vi "Begin.vi"(8 "error in":errorcluster) -> (0 "error out":errorcluster)   [LabVIEW 2019]
doc: "Called before other user functions, this VI is expected to open initial I/O refnums, load in file data, and do all program initialization. Notice that the <B>error out</B> terminal is simply used for data flow. Wiring it to other structures or subVIs ensures that this VI runs first."
uses:
  <vilib>/Rock Robotics/WPI/DriverStation/WPI_DriverStationRobotMode2.ctl
  Subsystems/Drive/Drive_Cluster.ctl
  Subsystems/Drive/Drive_States.ctl
  Subsystems/Intake/Intake_Cluster.ctl
  Subsystems/Intake/Intake_States.ctl
  Subsystems/Turret/Turret_Cluster.ctl
  Subsystems/Turret/Turret_States.ctl
  Subsystems/Magazine/Magazine_Cluster.ctl
  Subsystems/Magazine/Magazine_States.ctl
  Subsystems/Climb/Climb_Cluster.ctl
  Subsystems/Climb/Climb_States.ctl
  Subsystems/Control_Panel/Control_Panel_Cluster.ctl
  Subsystems/Control_Panel/Control_Panel_States.ctl
  <vilib>/Rock Robotics/WPI/Joystick/WPI_JoystickDeviceEnum.ctl
  <vilib>/Rock Robotics/WPI/ThirdParty/Phoenix-LabVIEW/Motor Controller/Controls/CTRE_Phoenix_MotorControl_ControlMode.ctl
  <vilib>/Rock Robotics/WPI/ThirdParty/REV Robotics/SPARK MAX/Typedef/Spark MAX Control Type.ctl
  Subsystems/Flywheel/Flywheel_Cluster.ctl
  Subsystems/Flywheel/Flywheel_States.ctl
  Robot Global Data.vi
  Globals/Drive_Globals.vi
  Globals/Intake_Globals.vi
  Globals/Turret_Globals.vi
  Globals/Magazine_Globals.vi
  Globals/Climb_Globals.vi
  Globals/Control_Panel_Globals.vi
  Globals/Joystick_Globals.vi
  Globals/Flywheel_Globals.vi
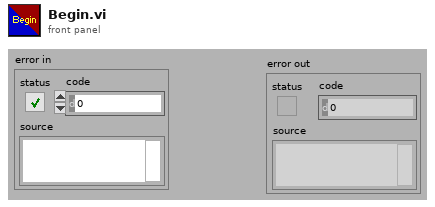
[diagram p1: front panel]
types:
  T1 = typedef "Spark MAX Control Type.ctl" = enum16{"Percent VBus", "Voltage", "Velocity", "Position", "Smart Motion", "Current", "Smart Velocity"}
  T2 = cluster{"P Gain":dbl, "I Gain":dbl, "D Gain":dbl, "F Gain":dbl, "I Zone":dbl, "Min Output":dbl, "Max Output":dbl}
  T3 = typedef "Flywheel_Cluster.ctl" = cluster{"Flywheel_Throttle":dbl, "Control_States":T4, "Auto_Speed":bool, "Flywheel_On":bool}
  T4 = typedef "Flywheel_States.ctl" = enum16{"No-Op", "Percent_Voltage", "Speed_Control_Manual", "Speed_Control_Auto"}
  T5 = typedef "CTRE_Phoenix_MotorControl_ControlMode.ctl" = u16
  T6 = typedef "WPI_JoystickDeviceEnum.ctl" = enum16{"USB 0", "USB 1", "USB 2", "USB 3", "USB 4", "USB 5"}
  T7 = typedef "Control_Panel_Cluster.ctl" = cluster{"Control_State":T8, "Start_Movement":bool, "Abort":bool, "Rotation_Control?":bool, "Positional_Control? ":bool, "Throttle":dbl}
  T8 = typedef "Control_Panel_States.ctl" = enum16{"No-Op", "Rotational_Control", "Positional_Control", "Manual_Control"}
  T9 = typedef "Climb_Cluster.ctl" = cluster{"Control_State":T10, "Extend_Climber?":bool, "Clamp?":bool, "Balance?":bool, "Transverse_Throttle":dbl, "Elevator_Throttle":dbl, "Control_Panel_Setpoint?":bool, "Auto-Balance":bool, "Pivot_Throttle":dbl}
  T10 = typedef "Climb_States.ctl" = enum16{"No-Op", "Extending", "Clamping", "Balancing", "Manual_Control"}
  T11 = typedef "Magazine_Cluster.ctl" = cluster{"Control_States":T12, "Fire":bool, "Magazine_Throttle":dbl}
  T12 = typedef "Magazine_States.ctl" = enum16{"No-Op", "Loading", "Fire", "Unjam", "Manual"}
  T13 = typedef "Turret_Cluster.ctl" = cluster{"Auto-Target?":bool, "Control_State":T14, "Turret_Spin_Speed":dbl, "Turret_Spin_Speed_Control?":bool}
  T14 = typedef "Turret_States.ctl" = enum16{"Manual_Percent_Voltage", "Manual_Speed_Control", "Auto-Target"}
  T15 = typedef "Intake_Cluster.ctl" = cluster{"Control_State":T16, "Intake_On":bool, "Intake_Extended":bool, "Intake_Throttle":dbl}
  T16 = typedef "Intake_States.ctl" = enum16{"Manual_Control"}
  T17 = typedef "Drive_Cluster.ctl" = cluster{"Control_State":T18, "Angular_Throttle":dbl, "Linear_Throttle":dbl, "Torque_Changing":bool}
  T18 = typedef "Drive_States.ctl" = enum16{"Percent_Voltage_Control", "Speed_Control"}
  T19 = typedef "WPI_DriverStationRobotMode2.ctl" = enum16{"Autonomous Disabled", "Autonomous Enabled", "Teleop Disabled", "Teleop Enabled", "Disconnected", "Finish", "Test Disabled", "Test Enabled", "Emergency Stopped"}
  T20 = typedef "WPI_JoystickDevRef.ctl" = cluster{"Device":T6}
  T21 = typedef "WPI_MotorControlDeviceRef.ctl" = cluster{"DeviceStatus":errorcluster, "Type":T22, "PWM":cluster{"PWM Channel":T23, "DeadBand":T24}, "CAN":cluster{"Device Number":u8, "SetOutput VI Ref":variant, "GetOutput VI Ref":variant, "Enable VI Ref":variant, "Disable VI Ref":variant, "Data":variant}, "Invert":bool, "DIO PWM":cluster{"PWM \"Enable\" Channel":T23, "DIOChannel":T25, "PWM Rate":dbl}}
  T22 = typedef "WPI_MotorControlType.ctl" = enum16{"PWM", "CAN", "DIO PWM"}
  T23 = typedef "FPGA_DIOPWMChannel.ctl" = enum8{"PWM 0", "PWM 1", "PWM 2", "PWM 3", "PWM 4", "PWM 5", "PWM 6", "PWM 7", "PWM 8", "PWM 9", "PWM MXP 0", "PWM MXP 1", "PWM MXP 2", "PWM MXP 3", "PWM MXP 4", "PWM MXP 5", "PWM MXP 6", "PWM MXP 7", "PWM MXP 8", "PWM MXP 9", "Invalid"}
  T24 = typedef "WPI_PWMDeadband.ctl" = cluster{"Name":string, "maxPositivePwm":i32, "minPositivePwm":i32, "centerPwm":i32, "maxNegativePwm":i32, "minNegativePwm":i32, "angularRange":u16}
  T25 = typedef "FPGA_DIOChannel.ctl" = enum8{"DIO 0", "DIO 1", "DIO 2", "DIO 3", "DIO 4", "DIO 5", "DIO 6", "DIO 7", "DIO 8", "DIO 9", "DIO MXP 0", "DIO MXP 1", "DIO MXP 2", "DIO MXP 3", "DIO MXP 4", "DIO MXP 5", "DIO MXP 6", "DIO MXP 7", "DIO MXP 8", "DIO MXP 9", "DIO MXP 10", "DIO MXP 11", "DIO MXP 12", "DIO MXP 13", "DIO MXP 14", "DIO MXP 15", "SPI Port CS1", "SPI Port CS2", "SPI Port CS3", "SPI Port MISO", "SPI Port MOSI", "Invalid"}
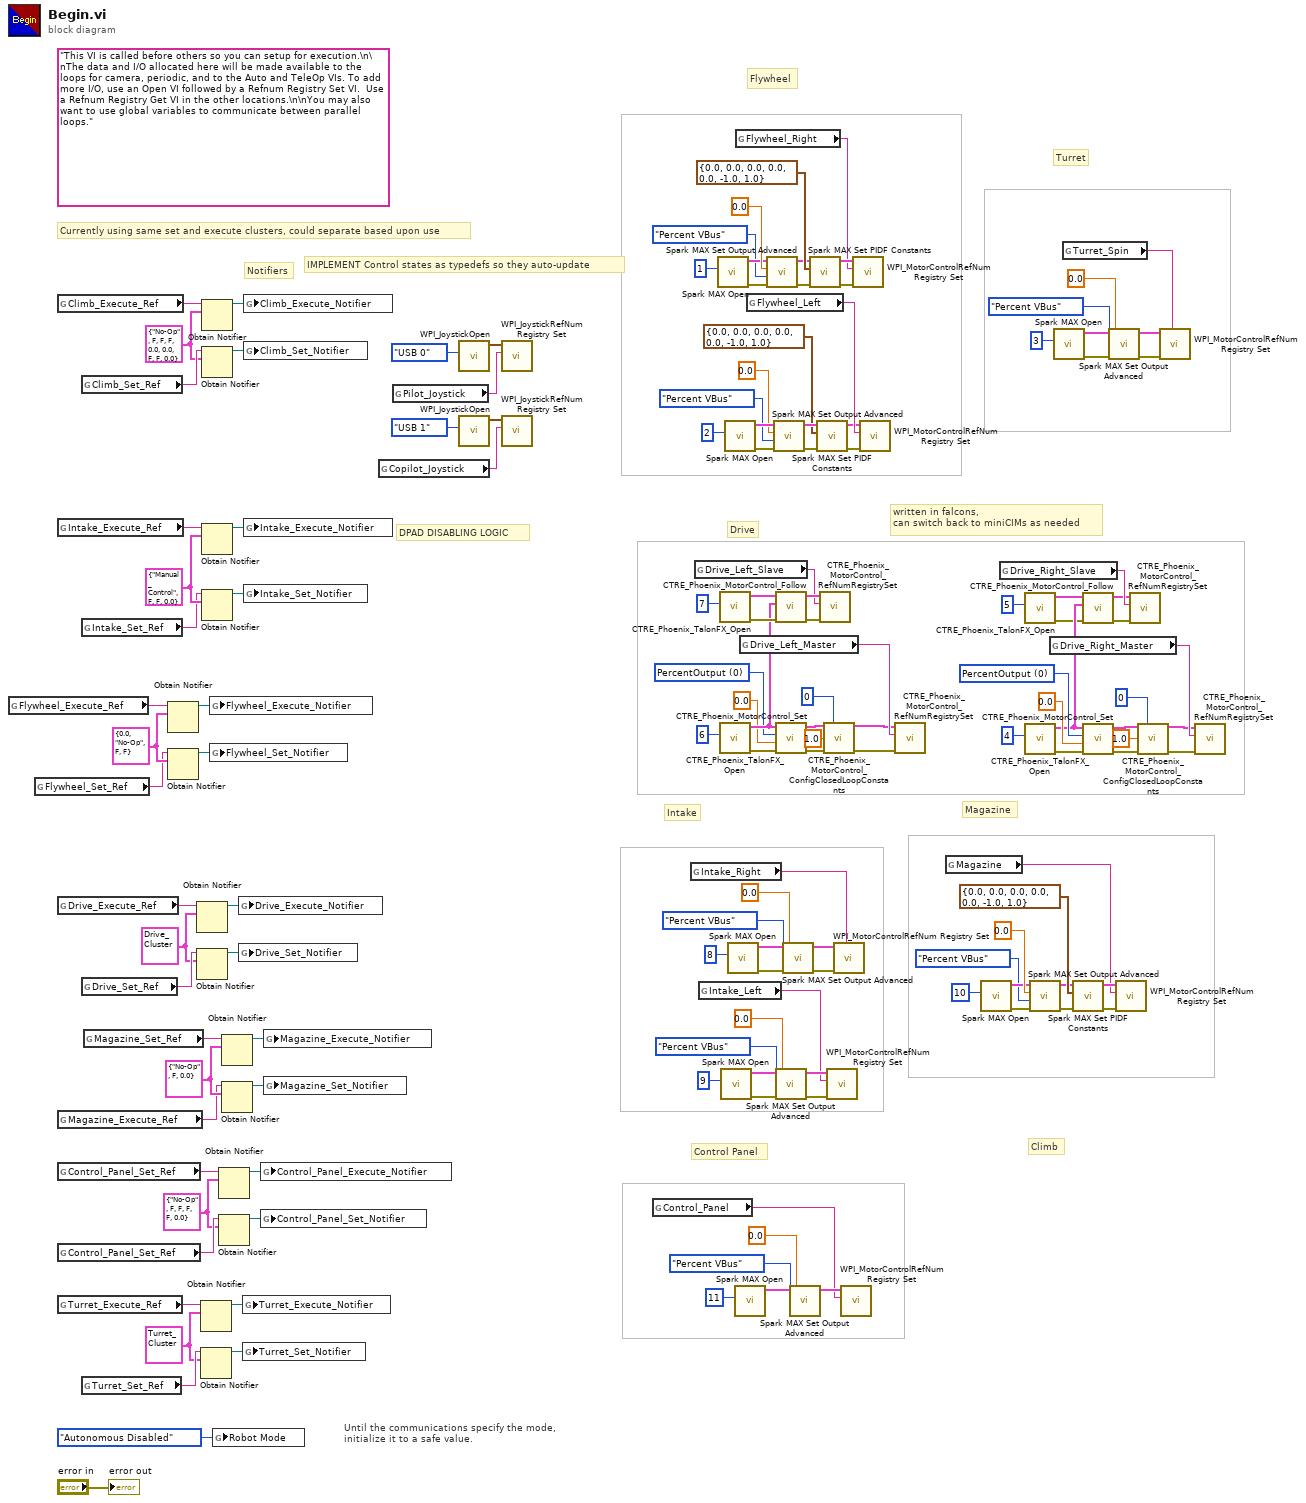
[diagram p0: block diagram]
diagram:
  w29 = T3 {"Flywheel_Throttle"=0.0, "Control_States"=enum."No-Op", "Auto_Speed"=FALSE, "Flywheel_On"=FALSE}
  w79 = T5 0 items=["PercentOutput"=0, "Position"=1, "Velocity"=2, "Current"=3, "Follower"=5, "MotionProfile"=6, "MotionMagic"=7, "MotionProfileArc"=10, "Disabled"=15] ("Control Mode")
  w95 = T5 0 items=["PercentOutput"=0, "Position"=1, "Velocity"=2, "Current"=3, "Follower"=5, "MotionProfile"=6, "MotionMagic"=7, "MotionProfileArc"=10, "Disabled"=15] ("Control Mode")
  w123 = T7 {"Control_State"=enum."No-Op", "Start_Movement"=FALSE, "Abort"=FALSE, "Rotation_Control?"=FALSE, "Positional_Control? "=FALSE, "Throttle"=0.0}
  w127 = T9 {"Control_State"=enum."No-Op", "Extend_Climber?"=FALSE, "Clamp?"=FALSE, "Balance?"=FALSE, "Transverse_Throttle"=0.0, "Elevator_Throttle"=0.0, "Control_Panel_Setpoint?"=FALSE, "Auto-Balance"=FALSE, "Pivot_Throttle"=0.0}
  w131 = T11 {"Control_States"=enum."No-Op", "Fire"=FALSE, "Magazine_Throttle"=0.0}
  w132 = T13 {"Auto-Target?"=FALSE, "Control_State"=enum."Manual_Percent_Voltage", "Turret_Spin_Speed"=0.0, "Turret_Spin_Speed_Control?"=FALSE}
  w137 = T15 {"Control_State"=enum."Manual_Control", "Intake_On"=FALSE, "Intake_Extended"=FALSE, "Intake_Throttle"=0.0}
  w138 = T17 {"Control_State"=enum."Percent_Voltage_Control", "Angular_Throttle"=0.0, "Linear_Throttle"=0.0, "Torque_Changing"=FALSE}
  (unwired) "This VI is called before others so you can setup for execution.\n\nThe data and I/O allocated here will be made available to the loops for camera, periodic, and to the Auto and TeleOp VIs. To add more I/O, use an Open VI followed by a Refnum Registry Set VI.  Use a Refnum Registry Get VI in the other locations.\n\nYou may also want to use global variables to communicate between parallel loops."
  # "Climb"
  # "Control Panel"
  # "Magazine"
  # "Intake"
  # "written in falcons, \ncan switch back to miniCIMs as needed"
  # "Drive"
  # "Turret"
  # "Flywheel"
  # "DPAD DISABLING LOGIC"
  # "IMPLEMENT Control states as typedefs so they auto-update"
  # "Notifiers"
  # "Currently using same set and execute clusters, could separate based upon use"
  # "Until the communications specify the mode,\ninitialize it to a safe value."
  n1 = global read "Flywheel_Globals.vi" "Flywheel_Execute_Ref"() -> (w28:string)
  n2 = global read "Flywheel_Globals.vi" "Flywheel_Set_Ref"() -> (w27:string)
  n3 = global read "Climb_Globals.vi" "Climb_Execute_Ref"() -> (w126:string)
  n4 = global read "Intake_Globals.vi" "Intake_Execute_Ref"() -> (w136:string)
  n5 = global read "Drive_Globals.vi" "Drive_Execute_Ref"() -> (w139:string)
  n6 = global read "Magazine_Globals.vi" "Magazine_Execute_Ref"() -> (w130:string)
  n7 = global read "Control_Panel_Globals.vi" "Control_Panel_Set_Ref"() -> (w125:string)
  n8 = global read "Control_Panel_Globals.vi" "Control_Panel_Set_Ref"() -> (w124:string)
  n9 = global read "Turret_Globals.vi" "Turret_Execute_Ref"() -> (w134:string)
  n10 = global read "Climb_Globals.vi" "Climb_Set_Ref"() -> (w128:string)
  n11 = global read "Intake_Globals.vi" "Intake_Set_Ref"() -> (w135:string)
  n12 = global read "Drive_Globals.vi" "Drive_Set_Ref"() -> (w140:string)
  n13 = global read "Turret_Globals.vi" "Turret_Set_Ref"() -> (w133:string)
  n14 = global read "Magazine_Globals.vi" "Magazine_Set_Ref"() -> (w129:string)
  n15 = Obtain Notifier(name (unnamed)=w28, notification data type=w29) -> (notifier out=w25:refnum<notifier>)  [unwired: 2 in, 2 out]
  n16 = Obtain Notifier(name (unnamed)=w27, notification data type=w29) -> (notifier out=w26:refnum<notifier>)  [unwired: 2 in, 2 out]
  n17 = Obtain Notifier(name (unnamed)=w139, notification data type=w138) -> (notifier out=w117:refnum<notifier>)  [unwired: 2 in, 2 out]
  n18 = Obtain Notifier(name (unnamed)=w140, notification data type=w138) -> (notifier out=w118:refnum<notifier>)  [unwired: 2 in, 2 out]
  n19 = Obtain Notifier(name (unnamed)=w134, notification data type=w132) -> (notifier out=w111:refnum<notifier>)  [unwired: 2 in, 2 out]
  n20 = Obtain Notifier(name (unnamed)=w133, notification data type=w132) -> (notifier out=w112:refnum<notifier>)  [unwired: 2 in, 2 out]
  n21 = Obtain Notifier(name (unnamed)=w126, notification data type=w127) -> (notifier out=w121:refnum<notifier>)  [unwired: 2 in, 2 out]
  n22 = Obtain Notifier(name (unnamed)=w128, notification data type=w127) -> (notifier out=w122:refnum<notifier>)  [unwired: 2 in, 2 out]
  n23 = Obtain Notifier(name (unnamed)=w136, notification data type=w137) -> (notifier out=w119:refnum<notifier>)  [unwired: 2 in, 2 out]
  n24 = Obtain Notifier(name (unnamed)=w135, notification data type=w137) -> (notifier out=w120:refnum<notifier>)  [unwired: 2 in, 2 out]
  n25 = global write "Flywheel_Globals.vi" "Flywheel_Execute_Notifier"(w25) -> ()
  n26 = global write "Flywheel_Globals.vi" "Flywheel_Set_Notifier"(w26) -> ()
  n27 = global write "Robot Global Data.vi" "Robot Mode"(WPI_DriverStationRobotMode2."Autonomous Disabled" ("Robot Mode")) -> ()
  n28 = Obtain Notifier(name (unnamed)=w125, notification data type=w123) -> (notifier out=w113:refnum<notifier>)  [unwired: 2 in, 2 out]
  n29 = Obtain Notifier(name (unnamed)=w124, notification data type=w123) -> (notifier out=w114:refnum<notifier>)  [unwired: 2 in, 2 out]
  n30 = Obtain Notifier(name (unnamed)=w129, notification data type=w131) -> (notifier out=w115:refnum<notifier>)  [unwired: 2 in, 2 out]
  n31 = Obtain Notifier(name (unnamed)=w130, notification data type=w131) -> (notifier out=w116:refnum<notifier>)  [unwired: 2 in, 2 out]
  n32 = global write "Drive_Globals.vi" "Drive_Execute_Notifier"(w117) -> ()
  n33 = global write "Drive_Globals.vi" "Drive_Set_Notifier"(w118) -> ()
  n34 = global write "Turret_Globals.vi" "Turret_Execute_Notifier"(w111) -> ()
  n35 = global write "Turret_Globals.vi" "Turret_Set_Notifier"(w112) -> ()
  n36 = global write "Climb_Globals.vi" "Climb_Execute_Notifier"(w121) -> ()
  n37 = global write "Climb_Globals.vi" "Climb_Set_Notifier"(w122) -> ()
  n38 = global write "Intake_Globals.vi" "Intake_Execute_Notifier"(w119) -> ()
  n39 = global write "Intake_Globals.vi" "Intake_Set_Notifier"(w120) -> ()
  n40 = global write "Control_Panel_Globals.vi" "Control_Panel_Execute_Notifier"(w113) -> ()
  n41 = global write "Control_Panel_Globals.vi" "Control_Panel_Set_Notifier"(w114) -> ()
  n42 = global write "Magazine_Globals.vi" "Magazine_Execute_Notifier"(w115) -> ()
  n43 = global write "Magazine_Globals.vi" "Magazine_Set_Notifier"(w116) -> ()
  n44 = global read "Joystick_Globals.vi" "Copilot_Joystick"() -> (w105:string)
  n45 = global read "Joystick_Globals.vi" "Pilot_Joystick"() -> (w106:string)
  n46 = call <vilib>:"WPI_JoystickOpen.vi"("JoystickDevice"=WPI_JoystickDeviceEnum."USB 0") -> ("JoystickDevRef"=w110:T20)  [unwired: 10 in]
  n47 = call <vilib>:"WPI_JoystickOpen.vi"("JoystickDevice"=WPI_JoystickDeviceEnum."USB 1") -> ("JoystickDevRef"=w109:T20)  [unwired: 10 in]
  n48 = call <vilib>:"WPI_JoystickRefNum Registry Set.vi"("refnum name"=w106, "JoystickDevRef"=w110) -> ()  [unwired: 8 in, 2 out]
  n49 = call <vilib>:"WPI_JoystickRefNum Registry Set.vi"("refnum name"=w105, "JoystickDevRef"=w109) -> ()  [unwired: 8 in, 2 out]
  n50 = global read "Control_Panel_Globals.vi" "Control_Panel"() -> (w1:string)
  n51 = global read "Intake_Globals.vi" "Intake_Right"() -> (w33:string)
  n52 = global read "Drive_Globals.vi" "Drive_Left_Slave"() -> (w77:string)
  n53 = global read "Intake_Globals.vi" "Intake_Left"() -> (w32:string)
  n54 = call <vilib>:"Spark MAX Open.vi"("Device Number"=u8 1) -> ("error out"=w13:errorcluster, "MotorControlDeviceRef"=w47:T21)  [unwired: 9 in]
  n55 = call <vilib>:"CTRE_Phoenix_TalonFX_Open.vi"("Device Number"=u8 7) -> ("error out"=w86:errorcluster, "CAN Talon SRX Ref"=w85:T21)  [unwired: 9 in]
  n56 = call <vilib>:"CTRE_Phoenix_TalonFX_Open.vi"("Device Number"=u8 6) -> ("error out"=w78:errorcluster, "CAN Talon SRX Ref"=w84:T21)  [unwired: 9 in]
  n57 = call <vilib>:"Spark MAX Open.vi"("Device Number"=u8 9) -> ("error out"=w31:errorcluster, "MotorControlDeviceRef"=w35:T21)  [unwired: 9 in]
  n58 = call <vilib>:"Spark MAX Open.vi"("Device Number"=u8 2) -> ("error out"=w103:errorcluster, "MotorControlDeviceRef"=w104:T21)  [unwired: 9 in]
  n59 = call <vilib>:"Spark MAX Open.vi"("Device Number"=u8 8) -> ("error out"=w42:errorcluster, "MotorControlDeviceRef"=w44:T21)  [unwired: 9 in]
  n60 = call <vilib>:"Spark MAX Open.vi"("Device Number"=u8 11) -> ("MotorControlDeviceRef"=w5:T21)  [unwired: 9 in, 1 out]
  n61 = global read "Flywheel_Globals.vi" "Flywheel_Right"() -> (w49:string)
  n62 = global read "Drive_Globals.vi" "Drive_Left_Master"() -> (w81:string)
  n63 = global read "Flywheel_Globals.vi" "Flywheel_Left"() -> (w101:string)
  n64 = call <vilib>:"Spark MAX Set Output Advanced.vi"("error in (no error)"=w13, "Control Mode"=Spark_MAX_Control_Type."Percent VBus", "Setpoint"=0.0, "MotorControlDevRef"=w47) -> ("error out"=w12:errorcluster, "MotorControlDevRef"=w51:T21)  [unwired: 6 in]
  n65 = call <vilib>:"Spark MAX Set Output Advanced.vi"("error in (no error)"=w103, "Control Mode"=Spark_MAX_Control_Type."Percent VBus", "Setpoint"=0.0, "MotorControlDevRef"=w104) -> ("error out"=w58:errorcluster, "MotorControlDevRef"=w57:T21)  [unwired: 6 in]
  n66 = call <vilib>:"CTRE_Phoenix_MotorControl_Follow.vi"("error in (no error)"=w86, "Master Controller to Follow"=w84, "PhoenixMotorControlDevRef"=w85) -> ("error out"=w83:errorcluster, "PhoenixMotorControlDevRef"=w82:T21)  [unwired: 7 in]
  n67 = call <vilib>:"CTRE_Phoenix_MotorControl_Set.vi"("error in (no error)"=w78, "Output"=0.0, "Control Mode"=w79, "PhoenixMotorControlDevRef"=w84) -> ("error out"=w71:errorcluster, "PhoenixMotorControlDevRef"=w72:T21)  [unwired: 6 in]
  n68 = call <vilib>:"Spark MAX Set Output Advanced.vi"("error in (no error)"=w31, "Control Mode"=Spark_MAX_Control_Type."Percent VBus", "Setpoint"=0.0, "MotorControlDevRef"=w35) -> ("error out"=w30:errorcluster, "MotorControlDevRef"=w36:T21)  [unwired: 6 in]
  n69 = call <vilib>:"Spark MAX Set Output Advanced.vi"("error in (no error)"=w42, "Control Mode"=Spark_MAX_Control_Type."Percent VBus", "Setpoint"=0.0, "MotorControlDevRef"=w44) -> ("error out"=w41:errorcluster, "MotorControlDevRef"=w43:T21)  [unwired: 6 in]
  n70 = call <vilib>:"Spark MAX Set Output Advanced.vi"("Control Mode"=Spark_MAX_Control_Type."Percent VBus", "Setpoint"=0.0, "MotorControlDevRef"=w5) -> ("MotorControlDevRef"=w4:T21)  [unwired: 7 in, 1 out]
  n71 = call <vilib>:"Spark MAX Set PIDF Constants.vi"("error in"=w12, "PID Constants"=T2 {"P Gain"=0.0, "I Gain"=0.0, "D Gain"=0.0, "F Gain"=0.0, "I Zone"=0.0, "Min Output"=-1.0, "Max Output"=1.0}, "MotorControlDeviceRef"=w51) -> ("error out"=w11:errorcluster, "MotorControlDeviceRef"=w52:T21)  [unwired: 7 in]
  n72 = call <vilib>:"Spark MAX Set PIDF Constants.vi"("error in"=w58, "PID Constants"=T2 {"P Gain"=0.0, "I Gain"=0.0, "D Gain"=0.0, "F Gain"=0.0, "I Zone"=0.0, "Min Output"=-1.0, "Max Output"=1.0}, "MotorControlDeviceRef"=w57) -> ("error out"=w56:errorcluster, "MotorControlDeviceRef"=w55:T21)  [unwired: 7 in]
  n73 = call <vilib>:"CTRE_Phoenix_MotorControl_RefNumRegistrySet.vi"("error in (no error)"=w83, "refnum name"=w77, "PhoenixMotorControlDevRef"=w82) -> ()  [unwired: 7 in, 2 out]
  n74 = call <vilib>:"CTRE_Phoenix_MotorControl_ConfigClosedLoopConstants.vi"("PhoenixMotorControlDevRef"=w72, "slotIdx"=0, "P"=1.0, "error in (no error)"=w71) -> ("PhoenixMotorControlDevRef"=w70:T21, "error out"=w69:errorcluster)  [unwired: 10 in]
  n75 = call <vilib>:"WPI_MotorControlRefNum Registry Set.vi"("error in (no error)"=w30, "refnum name"=w32, "MotorControlDevRef"=w36) -> ()  [unwired: 7 in, 2 out]
  n76 = call <vilib>:"WPI_MotorControlRefNum Registry Set.vi"("error in (no error)"=w41, "refnum name"=w33, "MotorControlDevRef"=w43) -> ()  [unwired: 7 in, 2 out]
  n77 = call <vilib>:"WPI_MotorControlRefNum Registry Set.vi"("refnum name"=w1, "MotorControlDevRef"=w4) -> ()  [unwired: 8 in, 2 out]
  n78 = call <vilib>:"WPI_MotorControlRefNum Registry Set.vi"("error in (no error)"=w11, "refnum name"=w49, "MotorControlDevRef"=w52) -> ()  [unwired: 7 in, 2 out]
  n79 = call <vilib>:"WPI_MotorControlRefNum Registry Set.vi"("error in (no error)"=w56, "refnum name"=w101, "MotorControlDevRef"=w55) -> ()  [unwired: 7 in, 2 out]
  n80 = call <vilib>:"CTRE_Phoenix_MotorControl_RefNumRegistrySet.vi"("error in (no error)"=w69, "refnum name"=w81, "PhoenixMotorControlDevRef"=w70) -> ()  [unwired: 7 in, 2 out]
  n81 = global read "Magazine_Globals.vi" "Magazine"() -> (w17:string)
  n82 = call <vilib>:"Spark MAX Open.vi"("Device Number"=u8 10) -> ("error out"=w16:errorcluster, "MotorControlDeviceRef"=w19:T21)  [unwired: 9 in]
  n83 = global read "Drive_Globals.vi" "Drive_Right_Slave"() -> (w92:string)
  n84 = call <vilib>:"CTRE_Phoenix_TalonFX_Open.vi"("Device Number"=u8 5) -> ("error out"=w87:errorcluster, "CAN Talon SRX Ref"=w88:T21)  [unwired: 9 in]
  n85 = call <vilib>:"CTRE_Phoenix_TalonFX_Open.vi"("Device Number"=u8 4) -> ("error out"=w96:errorcluster, "CAN Talon SRX Ref"=w89:T21)  [unwired: 9 in]
  n86 = call <vilib>:"Spark MAX Set Output Advanced.vi"("error in (no error)"=w16, "Control Mode"=Spark_MAX_Control_Type."Percent VBus", "Setpoint"=0.0, "MotorControlDevRef"=w19) -> ("error out"=w15:errorcluster, "MotorControlDevRef"=w22:T21)  [unwired: 6 in]
  n87 = global read "Drive_Globals.vi" "Drive_Right_Master"() -> (w93:string)
  n88 = call <vilib>:"Spark MAX Open.vi"("Device Number"=u8 3) -> ("error out"=w64:errorcluster, "MotorControlDeviceRef"=w99:T21)  [unwired: 9 in]
  n89 = global read "Turret_Globals.vi" "Turret_Spin"() -> (w97:string)
  n90 = call <vilib>:"Spark MAX Set PIDF Constants.vi"("error in"=w15, "PID Constants"=T2 {"P Gain"=0.0, "I Gain"=0.0, "D Gain"=0.0, "F Gain"=0.0, "I Zone"=0.0, "Min Output"=-1.0, "Max Output"=1.0}, "MotorControlDeviceRef"=w22) -> ("error out"=w14:errorcluster, "MotorControlDeviceRef"=w23:T21)  [unwired: 7 in]
  n91 = call <vilib>:"CTRE_Phoenix_MotorControl_Follow.vi"("error in (no error)"=w87, "Master Controller to Follow"=w89, "PhoenixMotorControlDevRef"=w88) -> ("error out"=w90:errorcluster, "PhoenixMotorControlDevRef"=w91:T21)  [unwired: 7 in]
  n92 = call <vilib>:"CTRE_Phoenix_MotorControl_Set.vi"("error in (no error)"=w96, "Output"=0.0, "Control Mode"=w95, "PhoenixMotorControlDevRef"=w89) -> ("error out"=w67:errorcluster, "PhoenixMotorControlDevRef"=w68:T21)  [unwired: 6 in]
  n93 = call <vilib>:"Spark MAX Set Output Advanced.vi"("error in (no error)"=w64, "Control Mode"=Spark_MAX_Control_Type."Percent VBus", "Setpoint"=0.0, "MotorControlDevRef"=w99) -> ("error out"=w63:errorcluster, "MotorControlDevRef"=w98:T21)  [unwired: 6 in]
  n94 = call <vilib>:"WPI_MotorControlRefNum Registry Set.vi"("error in (no error)"=w14, "refnum name"=w17, "MotorControlDevRef"=w23) -> ()  [unwired: 7 in, 2 out]
  n95 = call <vilib>:"CTRE_Phoenix_MotorControl_RefNumRegistrySet.vi"("error in (no error)"=w90, "refnum name"=w92, "PhoenixMotorControlDevRef"=w91) -> ()  [unwired: 7 in, 2 out]
  n96 = call <vilib>:"CTRE_Phoenix_MotorControl_ConfigClosedLoopConstants.vi"("PhoenixMotorControlDevRef"=w68, "slotIdx"=0, "I"=1.0 ("P"), "error in (no error)"=w67) -> ("PhoenixMotorControlDevRef"=w65:T21, "error out"=w66:errorcluster)  [unwired: 10 in]
  n97 = call <vilib>:"WPI_MotorControlRefNum Registry Set.vi"("error in (no error)"=w63, "refnum name"=w97, "MotorControlDevRef"=w98) -> ()  [unwired: 7 in, 2 out]
  n98 = call <vilib>:"CTRE_Phoenix_MotorControl_RefNumRegistrySet.vi"("error in (no error)"=w66, "refnum name"=w93, "PhoenixMotorControlDevRef"=w65) -> ()  [unwired: 7 in, 2 out]
  "error out" <- "error in"
